vi "rcvr text files to formated csv files Main VI.vi"() -> ()   [LabVIEW 2011]
uses:
  <vilib>/Utility/file.llb/Read From Spreadsheet File (string).vi
panel:
  in  "leap year":enum16{"NON Leap Year", "Leap Year"}(ring)
  in  "Directories to scan for all rcvr files":path[](array[path])
  in  "forced Elevation offset\n(Must by negative number)":dbl=-3.3537 max=0.0 format="%.4g"
  in  "Grennich Offset":dbl=-8.0
  out "stop time":timestamp
  out "start time":timestamp
  out "# of files already done":i32
  out "# of files to convert":i32
  in  "first part of CSV file name (date will be added to end of file)":string
  in  "Directory to save new CSV files into":path
  # "Use -8 for Pacific standard time. Correct from UTM time to Local Standard Time.\nThere is a VI that corrects for DST. (Only good for 2011)"
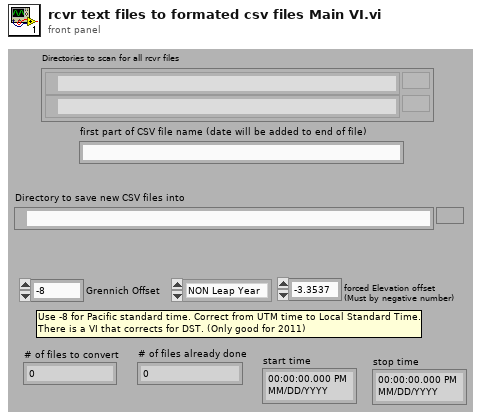
[diagram p1: front panel]
types:
  T1 = enum16{"open", "replace", "create", "open or create", "replace or create", "replace or create with confirmation"}
  T2 = cluster{"Time of NEMA":cluster{"Seconds":i32, "Minutes":i32, "Hours":i32}, "Lat-Long in Decimal Degrees":cluster{"Latitude (DD)":dbl, "Longitude (DD)":dbl}, "Point quality variables":cluster{"HDOP":dbl, "#Sats":dbl, "fixQuality":dbl}, "Elevations":cluster{"Elevation (Mean Sea Level)":dbl, "geodal separation":dbl, "Elevation (Height above Elipsode)":dbl}}
  T3 = cluster{"Latitude (DD)":dbl, "Longitude (DD)":dbl}
  T4 = cluster{"Seconds":i32, "Minutes":i32, "Hours":i32}
  T5 = typedef "LVDateTimeRec.ctl" = cluster{"fractional second":dbl, "second":i32, "minute":i32, "hour":i32, "day of month":i32, "month":i32, "year":i32, "day of week":i32, "day of year":i32, "DST":i32}
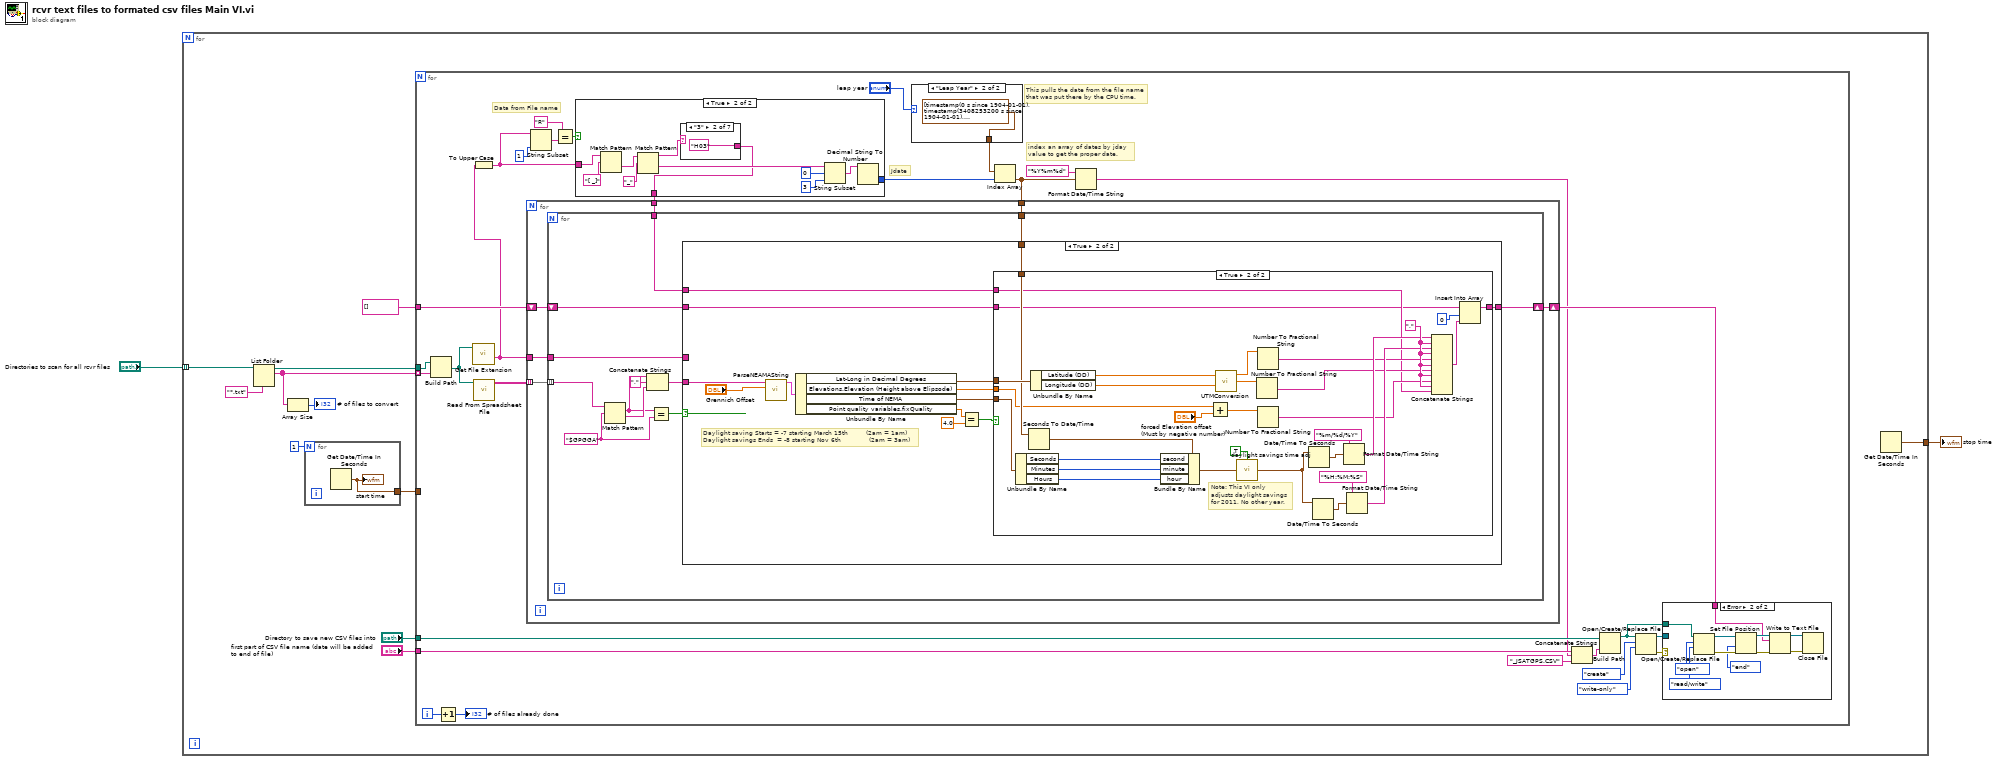
[diagram p0: block diagram]
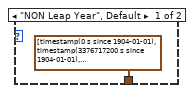
[diagram p2: hidden frame]
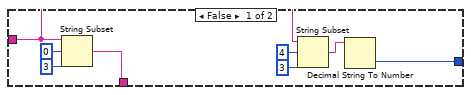
[diagram p3: hidden frame]
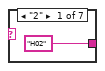
[diagram p4: hidden frame]
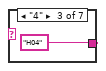
[diagram p5: hidden frame]
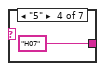
[diagram p6: hidden frame]
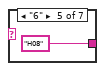
[diagram p7: hidden frame]
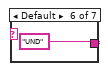
[diagram p8: hidden frame]
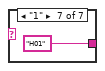
[diagram p9: hidden frame]
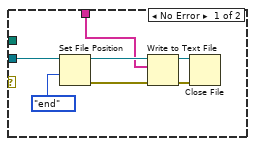
[diagram p10: hidden frame]
diagram:
  n1 = for {
    tunnel: [w4] -> w2
    tunnel: "Directories to scan for all rcvr files" -> [w3] mode=indexing
    n2 = List Folder(path=w3, pattern="*.txt") -> (path out=w12:path, filenames=w9:string[])  [unwired: 2 in, 2 out]
    n3 = Array Size(array=w9) -> (size(s)=→"# of files to convert":i32)
    n4 = for {
      N: 1 -> [_]
      tunnel: [w14] -> w6
      n5 = Get Date/Time In Seconds() -> (seconds since 1Jan1904=w14:timestamp)
      "start time" <- w14
    }
    n6 = for {
      tunnel: w12 -> [w44]
      tunnel: w9 -> [w43] mode=indexing
      tunnel: "Directory to save new CSV files into" -> [w39]
      tunnel: "first part of CSV file name (date will be added to end of file)" -> [w37]
      tunnel: string[] [] -> [w40]
      tunnel: w6 -> [_]
      i -> [w28]
      # "Jdate"
      # "This pulls the date from the file name\nthat was put there by the CPU time."
      # "Data from File name"
      # "index an array of dates by jday \nvalue to get the proper date."
      n7 = Build Path(base path=w44, name or relative path=w43) -> (appended path=w42:path)
      n8 = Increment(x=w28) -> (x+1=→"# of files already done":i32)
      n9 = call <vilib>:"Get File Extension.vi"("file"=w42) -> ("filename without extension"=w19:string)  [unwired: 7 in, 3 out]
      n10 = To Upper Case(1:w19) -> (0:w18:string)
      n11 = call-poly <vilib>:"Read From Spreadsheet File.vi"("file path (dialog if empty)"=w42) -> ("all rows"=w41:string[][])  [unwired: 6 in, 4 out]
      n12 = String Subset(string=w18, length (rest)=1 ("length (rest)")) -> (substring=w21:string)  [unwired: 1 in]
      n13 = Equal?(x="R", y=w21) -> (x = y?=w22:bool)
      n14 = case shown="True" w22 {
        tunnel: [w52 w58] -> w24
        tunnel: w18 -> [w48 w57]
        tunnel: [w47 w55] -> w16
        frame False {
          n15 = String Subset(string=w48, offset (0)=0, length (rest)=3 ("length (rest)")) -> (substring=w47:string)
          n16 = String Subset(string=w48, offset (0)=4, length (rest)=3 ("length (rest)")) -> (substring=w49:string)
          n17 = Decimal String To Number(string=w49) -> (number=w52:i32)  [unwired: 2 in, 1 out]
        }
        frame True {
          n18 = Match Pattern(string=w57, regular expression="[ _]") -> (after substring=w62:string)  [unwired: 1 in, 3 out]
          n19 = Match Pattern(string=w62, regular expression="_") -> (before substring=w56:string, after substring=w59:string)  [unwired: 1 in, 2 out]
          n20 = case shown="\"3\"" w56 {
            tunnel: ["H02" "H03" "H04" "H07" "H08" "UND" "H01"] -> w55
            frame "2" {
            }
            frame "3" {
            }
            frame "4" {
            }
            frame "5" {
            }
            frame "6" {
            }
            frame Default {
            }
            frame "1" {
            }
          }
          n21 = String Subset(string=w59, offset (0)=0, length (rest)=3 ("offset (0)")) -> (substring=w65:string)
          n22 = Decimal String To Number(string=w65) -> (number=w58:i32)  [unwired: 2 in, 1 out]
        }
      }
      n23 = case shown="\"Leap Year\"" "leap year" {
        tunnel: [timestamp[] [timestamp(0 s since 1904-01-01), timestamp(3376717200 s since 1904-01-01), timestamp(3376803600 s since 1904-01-01), timestamp(3376890000 s since 1904-01-01), timestamp(3376976400 s since 1904-01-01), timestamp(3377062800 s since 1904-01-01), timestamp(3377149200 s since 1904-01-01), timestamp(3377235600 s since 1904-01-01), timestamp(3377322000 s since 1904-01-01), timestamp(3377408400 s since 1904-01-01), timestamp(3377494800 s since 1904-01-01), timestamp(3377581200 s since 1904-01-01), timestamp(3377667600 s since 1904-01-01), timestamp(3377754000 s since 1904-01-01), timestamp(3377840400 s since 1904-01-01), timestamp(3377926800 s since 1904-01-01), timestamp(3378013200 s since 1904-01-01), timestamp(3378099600 s since 1904-01-01), timestamp(3378186000 s since 1904-01-01), timestamp(3378272400 s since 1904-01-01), timestamp(3378358800 s since 1904-01-01), timestamp(3378445200 s since 1904-01-01), timestamp(3378531600 s since 1904-01-01), timestamp(3378618000 s since 1904-01-01), timestamp(3378704400 s since 1904-01-01), timestamp(3378790800 s since 1904-01-01), timestamp(3378877200 s since 1904-01-01), timestamp(3378963600 s since 1904-01-01), timestamp(3379050000 s since 1904-01-01), timestamp(3379136400 s since 1904-01-01), timestamp(3379222800 s since 1904-01-01), timestamp(3379309200 s since 1904-01-01), timestamp(3379395600 s since 1904-01-01), timestamp(3379482000 s since 1904-01-01), timestamp(3379568400 s since 1904-01-01), timestamp(3379654800 s since 1904-01-01), timestamp(3379741200 s since 1904-01-01), timestamp(3379827600 s since 1904-01-01), timestamp(3379914000 s since 1904-01-01), timestamp(3380000400 s since 1904-01-01), timestamp(3380086800 s since 1904-01-01), timestamp(3380173200 s since 1904-01-01), timestamp(3380259600 s since 1904-01-01), timestamp(3380346000 s since 1904-01-01), timestamp(3380432400 s since 1904-01-01), timestamp(3380518800 s since 1904-01-01), timestamp(3380605200 s since 1904-01-01), timestamp(3380691600 s since 1904-01-01), timestamp(3380778000 s since 1904-01-01), timestamp(3380864400 s since 1904-01-01), timestamp(3380950800 s since 1904-01-01), timestamp(3381037200 s since 1904-01-01), timestamp(3381123600 s since 1904-01-01), timestamp(3381210000 s since 1904-01-01), timestamp(3381296400 s since 1904-01-01), timestamp(3381382800 s since 1904-01-01), timestamp(3381469200 s since 1904-01-01), timestamp(3381555600 s since 1904-01-01), timestamp(3381642000 s since 1904-01-01), timestamp(3381728400 s since 1904-01-01), timestamp(3381814800 s since 1904-01-01), timestamp(3381901200 s since 1904-01-01), timestamp(3381987600 s since 1904-01-01), timestamp(3382074000 s since 1904-01-01), timestamp(3382160400 s since 1904-01-01), timestamp(3382246800 s since 1904-01-01), timestamp(3382333200 s since 1904-01-01), timestamp(3382419600 s since 1904-01-01), timestamp(3382506000 s since 1904-01-01), timestamp(3382592400 s since 1904-01-01), timestamp(3382678800 s since 1904-01-01), timestamp(3382765200 s since 1904-01-01), timestamp(3382851600 s since 1904-01-01), timestamp(3382938000 s since 1904-01-01), timestamp(3383024400 s since 1904-01-01), timestamp(3383110800 s since 1904-01-01), timestamp(3383197200 s since 1904-01-01), timestamp(3383283600 s since 1904-01-01), timestamp(3383370000 s since 1904-01-01), timestamp(3383456400 s since 1904-01-01), timestamp(3383542800 s since 1904-01-01), timestamp(3383629200 s since 1904-01-01), timestamp(3383715600 s since 1904-01-01), timestamp(3383802000 s since 1904-01-01), timestamp(3383888400 s since 1904-01-01), timestamp(3383974800 s since 1904-01-01), timestamp(3384061200 s since 1904-01-01), timestamp(3384147600 s since 1904-01-01), timestamp(3384234000 s since 1904-01-01), timestamp(3384320400 s since 1904-01-01), timestamp(3384406800 s since 1904-01-01), timestamp(3384493200 s since 1904-01-01), timestamp(3384579600 s since 1904-01-01), timestamp(3384666000 s since 1904-01-01), timestamp(3384752400 s since 1904-01-01), timestamp(3384838800 s since 1904-01-01), timestamp(3384925200 s since 1904-01-01), timestamp(3385011600 s since 1904-01-01), timestamp(3385098000 s since 1904-01-01), timestamp(3385184400 s since 1904-01-01), timestamp(3385270800 s since 1904-01-01), timestamp(3385357200 s since 1904-01-01), timestamp(3385443600 s since 1904-01-01), timestamp(3385530000 s since 1904-01-01), timestamp(3385616400 s since 1904-01-01), timestamp(3385702800 s since 1904-01-01), timestamp(3385789200 s since 1904-01-01), timestamp(3385875600 s since 1904-01-01), timestamp(3385962000 s since 1904-01-01), timestamp(3386048400 s since 1904-01-01), timestamp(3386134800 s since 1904-01-01), timestamp(3386221200 s since 1904-01-01), timestamp(3386307600 s since 1904-01-01), timestamp(3386394000 s since 1904-01-01), timestamp(3386480400 s since 1904-01-01), timestamp(3386566800 s since 1904-01-01), timestamp(3386653200 s since 1904-01-01), timestamp(3386739600 s since 1904-01-01), timestamp(3386826000 s since 1904-01-01), timestamp(3386912400 s since 1904-01-01), timestamp(3386998800 s since 1904-01-01), timestamp(3387085200 s since 1904-01-01), timestamp(3387171600 s since 1904-01-01), timestamp(3387258000 s since 1904-01-01), timestamp(3387344400 s since 1904-01-01), timestamp(3387430800 s since 1904-01-01), timestamp(3387517200 s since 1904-01-01), timestamp(3387603600 s since 1904-01-01), timestamp(3387690000 s since 1904-01-01), timestamp(3387776400 s since 1904-01-01), timestamp(3387862800 s since 1904-01-01), timestamp(3387949200 s since 1904-01-01), timestamp(3388035600 s since 1904-01-01), timestamp(3388122000 s since 1904-01-01), timestamp(3388208400 s since 1904-01-01), timestamp(3388294800 s since 1904-01-01), timestamp(3388381200 s since 1904-01-01), timestamp(3388467600 s since 1904-01-01), timestamp(3388554000 s since 1904-01-01), timestamp(3388640400 s since 1904-01-01), timestamp(3388726800 s since 1904-01-01), timestamp(3388813200 s since 1904-01-01), timestamp(3388899600 s since 1904-01-01), timestamp(3388986000 s since 1904-01-01), timestamp(3389072400 s since 1904-01-01), timestamp(3389158800 s since 1904-01-01), timestamp(3389245200 s since 1904-01-01), timestamp(3389331600 s since 1904-01-01), timestamp(3389418000 s since 1904-01-01), timestamp(3389504400 s since 1904-01-01), timestamp(3389590800 s since 1904-01-01), timestamp(3389677200 s since 1904-01-01), timestamp(3389763600 s since 1904-01-01), timestamp(3389850000 s since 1904-01-01), timestamp(3389936400 s since 1904-01-01), timestamp(3390022800 s since 1904-01-01), timestamp(3390109200 s since 1904-01-01), timestamp(3390195600 s since 1904-01-01), timestamp(3390282000 s since 1904-01-01), timestamp(3390368400 s since 1904-01-01), timestamp(3390454800 s since 1904-01-01), timestamp(3390541200 s since 1904-01-01), timestamp(3390627600 s since 1904-01-01), timestamp(3390714000 s since 1904-01-01), timestamp(3390800400 s since 1904-01-01), timestamp(3390886800 s since 1904-01-01), timestamp(3390973200 s since 1904-01-01), timestamp(3391059600 s since 1904-01-01), timestamp(3391146000 s since 1904-01-01), timestamp(3391232400 s since 1904-01-01), timestamp(3391318800 s since 1904-01-01), timestamp(3391405200 s since 1904-01-01), timestamp(3391491600 s since 1904-01-01), timestamp(3391578000 s since 1904-01-01), timestamp(3391664400 s since 1904-01-01), timestamp(3391750800 s since 1904-01-01), timestamp(3391837200 s since 1904-01-01), timestamp(3391923600 s since 1904-01-01), timestamp(3392010000 s since 1904-01-01), timestamp(3392096400 s since 1904-01-01), timestamp(3392182800 s since 1904-01-01), timestamp(3392269200 s since 1904-01-01), timestamp(3392355600 s since 1904-01-01), timestamp(3392442000 s since 1904-01-01), timestamp(3392528400 s since 1904-01-01), timestamp(3392614800 s since 1904-01-01), timestamp(3392701200 s since 1904-01-01), timestamp(3392787600 s since 1904-01-01), timestamp(3392874000 s since 1904-01-01), timestamp(3392960400 s since 1904-01-01), timestamp(3393046800 s since 1904-01-01), timestamp(3393133200 s since 1904-01-01), timestamp(3393219600 s since 1904-01-01), timestamp(3393306000 s since 1904-01-01), timestamp(3393392400 s since 1904-01-01), timestamp(3393478800 s since 1904-01-01), timestamp(3393565200 s since 1904-01-01), timestamp(3393651600 s since 1904-01-01), timestamp(3393738000 s since 1904-01-01), timestamp(3393824400 s since 1904-01-01), timestamp(3393910800 s since 1904-01-01), timestamp(3393997200 s since 1904-01-01), timestamp(3394083600 s since 1904-01-01), timestamp(3394170000 s since 1904-01-01), timestamp(3394256400 s since 1904-01-01), timestamp(3394342800 s since 1904-01-01), timestamp(3394429200 s since 1904-01-01), timestamp(3394515600 s since 1904-01-01), timestamp(3394602000 s since 1904-01-01), timestamp(3394688400 s since 1904-01-01), timestamp(3394774800 s since 1904-01-01), timestamp(3394861200 s since 1904-01-01), timestamp(3394947600 s since 1904-01-01), timestamp(3395034000 s since 1904-01-01), timestamp(3395120400 s since 1904-01-01), timestamp(3395206800 s since 1904-01-01), timestamp(3395293200 s since 1904-01-01), timestamp(3395379600 s since 1904-01-01), timestamp(3395466000 s since 1904-01-01), timestamp(3395552400 s since 1904-01-01), timestamp(3395638800 s since 1904-01-01), timestamp(3395725200 s since 1904-01-01), timestamp(3395811600 s since 1904-01-01), timestamp(3395898000 s since 1904-01-01), timestamp(3395984400 s since 1904-01-01), timestamp(3396070800 s since 1904-01-01), timestamp(3396157200 s since 1904-01-01), timestamp(3396243600 s since 1904-01-01), timestamp(3396330000 s since 1904-01-01), timestamp(3396416400 s since 1904-01-01), timestamp(3396502800 s since 1904-01-01), timestamp(3396589200 s since 1904-01-01), timestamp(3396675600 s since 1904-01-01), timestamp(3396762000 s since 1904-01-01), timestamp(3396848400 s since 1904-01-01), timestamp(3396934800 s since 1904-01-01), timestamp(3397021200 s since 1904-01-01), timestamp(3397107600 s since 1904-01-01), timestamp(3397194000 s since 1904-01-01), timestamp(3397280400 s since 1904-01-01), timestamp(3397366800 s since 1904-01-01), timestamp(3397453200 s since 1904-01-01), timestamp(3397539600 s since 1904-01-01), timestamp(3397626000 s since 1904-01-01), timestamp(3397712400 s since 1904-01-01), timestamp(3397798800 s since 1904-01-01), timestamp(3397885200 s since 1904-01-01), timestamp(3397971600 s since 1904-01-01), timestamp(3398058000 s since 1904-01-01), timestamp(3398144400 s since 1904-01-01), timestamp(3398230800 s since 1904-01-01), timestamp(3398317200 s since 1904-01-01), timestamp(3398403600 s since 1904-01-01), timestamp(3398490000 s since 1904-01-01), timestamp(3398576400 s since 1904-01-01), timestamp(3398662800 s since 1904-01-01), timestamp(3398749200 s since 1904-01-01), timestamp(3398835600 s since 1904-01-01), timestamp(3398922000 s since 1904-01-01), timestamp(3399008400 s since 1904-01-01), timestamp(3399094800 s since 1904-01-01), timestamp(3399181200 s since 1904-01-01), timestamp(3399267600 s since 1904-01-01), timestamp(3399354000 s since 1904-01-01), timestamp(3399440400 s since 1904-01-01), timestamp(3399526800 s since 1904-01-01), timestamp(3399613200 s since 1904-01-01), timestamp(3399699600 s since 1904-01-01), timestamp(3399786000 s since 1904-01-01), timestamp(3399872400 s since 1904-01-01), timestamp(3399958800 s since 1904-01-01), timestamp(3400045200 s since 1904-01-01), timestamp(3400131600 s since 1904-01-01), timestamp(3400218000 s since 1904-01-01), timestamp(3400304400 s since 1904-01-01), timestamp(3400390800 s since 1904-01-01), timestamp(3400477200 s since 1904-01-01), timestamp(3400563600 s since 1904-01-01), timestamp(3400650000 s since 1904-01-01), timestamp(3400736400 s since 1904-01-01), timestamp(3400822800 s since 1904-01-01), timestamp(3400909200 s since 1904-01-01), timestamp(3400995600 s since 1904-01-01), timestamp(3401082000 s since 1904-01-01), timestamp(3401168400 s since 1904-01-01), timestamp(3401254800 s since 1904-01-01), timestamp(3401341200 s since 1904-01-01), timestamp(3401427600 s since 1904-01-01), timestamp(3401514000 s since 1904-01-01), timestamp(3401600400 s since 1904-01-01), timestamp(3401686800 s since 1904-01-01), timestamp(3401773200 s since 1904-01-01), timestamp(3401859600 s since 1904-01-01), timestamp(3401946000 s since 1904-01-01), timestamp(3402032400 s since 1904-01-01), timestamp(3402118800 s since 1904-01-01), timestamp(3402205200 s since 1904-01-01), timestamp(3402291600 s since 1904-01-01), timestamp(3402378000 s since 1904-01-01), timestamp(3402464400 s since 1904-01-01), timestamp(3402550800 s since 1904-01-01), timestamp(3402637200 s since 1904-01-01), timestamp(3402723600 s since 1904-01-01), timestamp(3402810000 s since 1904-01-01), timestamp(3402896400 s since 1904-01-01), timestamp(3402982800 s since 1904-01-01), timestamp(3403069200 s since 1904-01-01), timestamp(3403155600 s since 1904-01-01), timestamp(3403242000 s since 1904-01-01), timestamp(3403328400 s since 1904-01-01), timestamp(3403414800 s since 1904-01-01), timestamp(3403501200 s since 1904-01-01), timestamp(3403587600 s since 1904-01-01), timestamp(3403674000 s since 1904-01-01), timestamp(3403760400 s since 1904-01-01), timestamp(3403846800 s since 1904-01-01), timestamp(3403933200 s since 1904-01-01), timestamp(3404019600 s since 1904-01-01), timestamp(3404106000 s since 1904-01-01), timestamp(3404192400 s since 1904-01-01), timestamp(3404278800 s since 1904-01-01), timestamp(3404365200 s since 1904-01-01), timestamp(3404451600 s since 1904-01-01), timestamp(3404538000 s since 1904-01-01), timestamp(3404624400 s since 1904-01-01), timestamp(3404710800 s since 1904-01-01), timestamp(3404797200 s since 1904-01-01), timestamp(3404883600 s since 1904-01-01), timestamp(3404970000 s since 1904-01-01), timestamp(3405056400 s since 1904-01-01), timestamp(3405142800 s since 1904-01-01), timestamp(3405229200 s since 1904-01-01), timestamp(3405315600 s since 1904-01-01), timestamp(3405402000 s since 1904-01-01), timestamp(3405488400 s since 1904-01-01), timestamp(3405574800 s since 1904-01-01), timestamp(3405661200 s since 1904-01-01), timestamp(3405747600 s since 1904-01-01), timestamp(3405834000 s since 1904-01-01), timestamp(3405920400 s since 1904-01-01), timestamp(3406006800 s since 1904-01-01), timestamp(3406093200 s since 1904-01-01), timestamp(3406179600 s since 1904-01-01), timestamp(3406266000 s since 1904-01-01), timestamp(3406352400 s since 1904-01-01), timestamp(3406438800 s since 1904-01-01), timestamp(3406525200 s since 1904-01-01), timestamp(3406611600 s since 1904-01-01), timestamp(3406698000 s since 1904-01-01), timestamp(3406784400 s since 1904-01-01), timestamp(3406870800 s since 1904-01-01), timestamp(3406957200 s since 1904-01-01), timestamp(3407043600 s since 1904-01-01), timestamp(3407130000 s since 1904-01-01), timestamp(3407216400 s since 1904-01-01), timestamp(3407302800 s since 1904-01-01), timestamp(3407389200 s since 1904-01-01), timestamp(3407475600 s since 1904-01-01), timestamp(3407562000 s since 1904-01-01), timestamp(3407648400 s since 1904-01-01), timestamp(3407734800 s since 1904-01-01), timestamp(3407821200 s since 1904-01-01), timestamp(3407907600 s since 1904-01-01), timestamp(3407994000 s since 1904-01-01), timestamp(3408080400 s since 1904-01-01), timestamp(3408166800 s since 1904-01-01)] ("Julian day to calander day non leap year (index = Julian day)") timestamp[] [timestamp(0 s since 1904-01-01), timestamp(3408253200 s since 1904-01-01), timestamp(3408339600 s since 1904-01-01), timestamp(3408426000 s since 1904-01-01), timestamp(3408512400 s since 1904-01-01), timestamp(3408598800 s since 1904-01-01), timestamp(3408685200 s since 1904-01-01), timestamp(3408771600 s since 1904-01-01), timestamp(3408858000 s since 1904-01-01), timestamp(3408944400 s since 1904-01-01), timestamp(3409030800 s since 1904-01-01), timestamp(3409117200 s since 1904-01-01), timestamp(3409203600 s since 1904-01-01), timestamp(3409290000 s since 1904-01-01), timestamp(3409376400 s since 1904-01-01), timestamp(3409462800 s since 1904-01-01), timestamp(3409549200 s since 1904-01-01), timestamp(3409635600 s since 1904-01-01), timestamp(3409722000 s since 1904-01-01), timestamp(3409808400 s since 1904-01-01), timestamp(3409894800 s since 1904-01-01), timestamp(3409981200 s since 1904-01-01), timestamp(3410067600 s since 1904-01-01), timestamp(3410154000 s since 1904-01-01), timestamp(3410240400 s since 1904-01-01), timestamp(3410326800 s since 1904-01-01), timestamp(3410413200 s since 1904-01-01), timestamp(3410499600 s since 1904-01-01), timestamp(3410586000 s since 1904-01-01), timestamp(3410672400 s since 1904-01-01), timestamp(3410758800 s since 1904-01-01), timestamp(3410845200 s since 1904-01-01), timestamp(3410931600 s since 1904-01-01), timestamp(3411018000 s since 1904-01-01), timestamp(3411104400 s since 1904-01-01), timestamp(3411190800 s since 1904-01-01), timestamp(3411277200 s since 1904-01-01), timestamp(3411363600 s since 1904-01-01), timestamp(3411450000 s since 1904-01-01), timestamp(3411536400 s since 1904-01-01), timestamp(3411622800 s since 1904-01-01), timestamp(3411709200 s since 1904-01-01), timestamp(3411795600 s since 1904-01-01), timestamp(3411882000 s since 1904-01-01), timestamp(3411968400 s since 1904-01-01), timestamp(3412054800 s since 1904-01-01), timestamp(3412141200 s since 1904-01-01), timestamp(3412227600 s since 1904-01-01), timestamp(3412314000 s since 1904-01-01), timestamp(3412400400 s since 1904-01-01), timestamp(3412486800 s since 1904-01-01), timestamp(3412573200 s since 1904-01-01), timestamp(3412659600 s since 1904-01-01), timestamp(3412746000 s since 1904-01-01), timestamp(3412832400 s since 1904-01-01), timestamp(3412918800 s since 1904-01-01), timestamp(3413005200 s since 1904-01-01), timestamp(3413091600 s since 1904-01-01), timestamp(3413178000 s since 1904-01-01), timestamp(3413264400 s since 1904-01-01), timestamp(3413350800 s since 1904-01-01), timestamp(3413437200 s since 1904-01-01), timestamp(3413523600 s since 1904-01-01), timestamp(3413610000 s since 1904-01-01), timestamp(3413696400 s since 1904-01-01), timestamp(3413782800 s since 1904-01-01), timestamp(3413869200 s since 1904-01-01), timestamp(3413955600 s since 1904-01-01), timestamp(3414042000 s since 1904-01-01), timestamp(3414128400 s since 1904-01-01), timestamp(3414214800 s since 1904-01-01), timestamp(3414301200 s since 1904-01-01), timestamp(3414387600 s since 1904-01-01), timestamp(3414474000 s since 1904-01-01), timestamp(3414560400 s since 1904-01-01), timestamp(3414646800 s since 1904-01-01), timestamp(3414733200 s since 1904-01-01), timestamp(3414819600 s since 1904-01-01), timestamp(3414906000 s since 1904-01-01), timestamp(3414992400 s since 1904-01-01), timestamp(3415078800 s since 1904-01-01), timestamp(3415165200 s since 1904-01-01), timestamp(3415251600 s since 1904-01-01), timestamp(3415338000 s since 1904-01-01), timestamp(3415424400 s since 1904-01-01), timestamp(3415510800 s since 1904-01-01), timestamp(3415597200 s since 1904-01-01), timestamp(3415683600 s since 1904-01-01), timestamp(3415770000 s since 1904-01-01), timestamp(3415856400 s since 1904-01-01), timestamp(3415942800 s since 1904-01-01), timestamp(3416029200 s since 1904-01-01), timestamp(3416115600 s since 1904-01-01), timestamp(3416202000 s since 1904-01-01), timestamp(3416288400 s since 1904-01-01), timestamp(3416374800 s since 1904-01-01), timestamp(3416461200 s since 1904-01-01), timestamp(3416547600 s since 1904-01-01), timestamp(3416634000 s since 1904-01-01), timestamp(3416720400 s since 1904-01-01), timestamp(3416806800 s since 1904-01-01), timestamp(3416893200 s since 1904-01-01), timestamp(3416979600 s since 1904-01-01), timestamp(3417066000 s since 1904-01-01), timestamp(3417152400 s since 1904-01-01), timestamp(3417238800 s since 1904-01-01), timestamp(3417325200 s since 1904-01-01), timestamp(3417411600 s since 1904-01-01), timestamp(3417498000 s since 1904-01-01), timestamp(3417584400 s since 1904-01-01), timestamp(3417670800 s since 1904-01-01), timestamp(3417757200 s since 1904-01-01), timestamp(3417843600 s since 1904-01-01), timestamp(3417930000 s since 1904-01-01), timestamp(3418016400 s since 1904-01-01), timestamp(3418102800 s since 1904-01-01), timestamp(3418189200 s since 1904-01-01), timestamp(3418275600 s since 1904-01-01), timestamp(3418362000 s since 1904-01-01), timestamp(3418448400 s since 1904-01-01), timestamp(3418534800 s since 1904-01-01), timestamp(3418621200 s since 1904-01-01), timestamp(3418707600 s since 1904-01-01), timestamp(3418794000 s since 1904-01-01), timestamp(3418880400 s since 1904-01-01), timestamp(3418966800 s since 1904-01-01), timestamp(3419053200 s since 1904-01-01), timestamp(3419139600 s since 1904-01-01), timestamp(3419226000 s since 1904-01-01), timestamp(3419312400 s since 1904-01-01), timestamp(3419398800 s since 1904-01-01), timestamp(3419485200 s since 1904-01-01), timestamp(3419571600 s since 1904-01-01), timestamp(3419658000 s since 1904-01-01), timestamp(3419744400 s since 1904-01-01), timestamp(3419830800 s since 1904-01-01), timestamp(3419917200 s since 1904-01-01), timestamp(3420003600 s since 1904-01-01), timestamp(3420090000 s since 1904-01-01), timestamp(3420176400 s since 1904-01-01), timestamp(3420262800 s since 1904-01-01), timestamp(3420349200 s since 1904-01-01), timestamp(3420435600 s since 1904-01-01), timestamp(3420522000 s since 1904-01-01), timestamp(3420608400 s since 1904-01-01), timestamp(3420694800 s since 1904-01-01), timestamp(3420781200 s since 1904-01-01), timestamp(3420867600 s since 1904-01-01), timestamp(3420954000 s since 1904-01-01), timestamp(3421040400 s since 1904-01-01), timestamp(3421126800 s since 1904-01-01), timestamp(3421213200 s since 1904-01-01), timestamp(3421299600 s since 1904-01-01), timestamp(3421386000 s since 1904-01-01), timestamp(3421472400 s since 1904-01-01), timestamp(3421558800 s since 1904-01-01), timestamp(3421645200 s since 1904-01-01), timestamp(3421731600 s since 1904-01-01), timestamp(3421818000 s since 1904-01-01), timestamp(3421904400 s since 1904-01-01), timestamp(3421990800 s since 1904-01-01), timestamp(3422077200 s since 1904-01-01), timestamp(3422163600 s since 1904-01-01), timestamp(3422250000 s since 1904-01-01), timestamp(3422336400 s since 1904-01-01), timestamp(3422422800 s since 1904-01-01), timestamp(3422509200 s since 1904-01-01), timestamp(3422595600 s since 1904-01-01), timestamp(3422682000 s since 1904-01-01), timestamp(3422768400 s since 1904-01-01), timestamp(3422854800 s since 1904-01-01), timestamp(3422941200 s since 1904-01-01), timestamp(3423027600 s since 1904-01-01), timestamp(3423114000 s since 1904-01-01), timestamp(3423200400 s since 1904-01-01), timestamp(3423286800 s since 1904-01-01), timestamp(3423373200 s since 1904-01-01), timestamp(3423459600 s since 1904-01-01), timestamp(3423546000 s since 1904-01-01), timestamp(3423632400 s since 1904-01-01), timestamp(3423718800 s since 1904-01-01), timestamp(3423805200 s since 1904-01-01), timestamp(3423891600 s since 1904-01-01), timestamp(3423978000 s since 1904-01-01), timestamp(3424064400 s since 1904-01-01), timestamp(3424150800 s since 1904-01-01), timestamp(3424237200 s since 1904-01-01), timestamp(3424323600 s since 1904-01-01), timestamp(3424410000 s since 1904-01-01), timestamp(3424496400 s since 1904-01-01), timestamp(3424582800 s since 1904-01-01), timestamp(3424669200 s since 1904-01-01), timestamp(3424755600 s since 1904-01-01), timestamp(3424842000 s since 1904-01-01), timestamp(3424928400 s since 1904-01-01), timestamp(3425014800 s since 1904-01-01), timestamp(3425101200 s since 1904-01-01), timestamp(3425187600 s since 1904-01-01), timestamp(3425274000 s since 1904-01-01), timestamp(3425360400 s since 1904-01-01), timestamp(3425446800 s since 1904-01-01), timestamp(3425533200 s since 1904-01-01), timestamp(3425619600 s since 1904-01-01), timestamp(3425706000 s since 1904-01-01), timestamp(3425792400 s since 1904-01-01), timestamp(3425878800 s since 1904-01-01), timestamp(3425965200 s since 1904-01-01), timestamp(3426051600 s since 1904-01-01), timestamp(3426138000 s since 1904-01-01), timestamp(3426224400 s since 1904-01-01), timestamp(3426310800 s since 1904-01-01), timestamp(3426397200 s since 1904-01-01), timestamp(3426483600 s since 1904-01-01), timestamp(3426570000 s since 1904-01-01), timestamp(3426656400 s since 1904-01-01), timestamp(3426742800 s since 1904-01-01), timestamp(3426829200 s since 1904-01-01), timestamp(3426915600 s since 1904-01-01), timestamp(3427002000 s since 1904-01-01), timestamp(3427088400 s since 1904-01-01), timestamp(3427174800 s since 1904-01-01), timestamp(3427261200 s since 1904-01-01), timestamp(3427347600 s since 1904-01-01), timestamp(3427434000 s since 1904-01-01), timestamp(3427520400 s since 1904-01-01), timestamp(3427606800 s since 1904-01-01), timestamp(3427693200 s since 1904-01-01), timestamp(3427779600 s since 1904-01-01), timestamp(3427866000 s since 1904-01-01), timestamp(3427952400 s since 1904-01-01), timestamp(3428038800 s since 1904-01-01), timestamp(3428125200 s since 1904-01-01), timestamp(3428211600 s since 1904-01-01), timestamp(3428298000 s since 1904-01-01), timestamp(3428384400 s since 1904-01-01), timestamp(3428470800 s since 1904-01-01), timestamp(3428557200 s since 1904-01-01), timestamp(3428643600 s since 1904-01-01), timestamp(3428730000 s since 1904-01-01), timestamp(3428816400 s since 1904-01-01), timestamp(3428902800 s since 1904-01-01), timestamp(3428989200 s since 1904-01-01), timestamp(3429075600 s since 1904-01-01), timestamp(3429162000 s since 1904-01-01), timestamp(3429248400 s since 1904-01-01), timestamp(3429334800 s since 1904-01-01), timestamp(3429421200 s since 1904-01-01), timestamp(3429507600 s since 1904-01-01), timestamp(3429594000 s since 1904-01-01), timestamp(3429680400 s since 1904-01-01), timestamp(3429766800 s since 1904-01-01), timestamp(3429853200 s since 1904-01-01), timestamp(3429939600 s since 1904-01-01), timestamp(3430026000 s since 1904-01-01), timestamp(3430112400 s since 1904-01-01), timestamp(3430198800 s since 1904-01-01), timestamp(3430285200 s since 1904-01-01), timestamp(3430371600 s since 1904-01-01), timestamp(3430458000 s since 1904-01-01), timestamp(3430544400 s since 1904-01-01), timestamp(3430630800 s since 1904-01-01), timestamp(3430717200 s since 1904-01-01), timestamp(3430803600 s since 1904-01-01), timestamp(3430890000 s since 1904-01-01), timestamp(3430976400 s since 1904-01-01), timestamp(3431062800 s since 1904-01-01), timestamp(3431149200 s since 1904-01-01), timestamp(3431235600 s since 1904-01-01), timestamp(3431322000 s since 1904-01-01), timestamp(3431408400 s since 1904-01-01), timestamp(3431494800 s since 1904-01-01), timestamp(3431581200 s since 1904-01-01), timestamp(3431667600 s since 1904-01-01), timestamp(3431754000 s since 1904-01-01), timestamp(3431840400 s since 1904-01-01), timestamp(3431926800 s since 1904-01-01), timestamp(3432013200 s since 1904-01-01), timestamp(3432099600 s since 1904-01-01), timestamp(3432186000 s since 1904-01-01), timestamp(3432272400 s since 1904-01-01), timestamp(3432358800 s since 1904-01-01), timestamp(3432445200 s since 1904-01-01), timestamp(3432531600 s since 1904-01-01), timestamp(3432618000 s since 1904-01-01), timestamp(3432704400 s since 1904-01-01), timestamp(3432790800 s since 1904-01-01), timestamp(3432877200 s since 1904-01-01), timestamp(3432963600 s since 1904-01-01), timestamp(3433050000 s since 1904-01-01), timestamp(3433136400 s since 1904-01-01), timestamp(3433222800 s since 1904-01-01), timestamp(3433309200 s since 1904-01-01), timestamp(3433395600 s since 1904-01-01), timestamp(3433482000 s since 1904-01-01), timestamp(3433568400 s since 1904-01-01), timestamp(3433654800 s since 1904-01-01), timestamp(3433741200 s since 1904-01-01), timestamp(3433827600 s since 1904-01-01), timestamp(3433914000 s since 1904-01-01), timestamp(3434000400 s since 1904-01-01), timestamp(3434086800 s since 1904-01-01), timestamp(3434173200 s since 1904-01-01), timestamp(3434259600 s since 1904-01-01), timestamp(3434346000 s since 1904-01-01), timestamp(3434432400 s since 1904-01-01), timestamp(3434518800 s since 1904-01-01), timestamp(3434605200 s since 1904-01-01), timestamp(3434691600 s since 1904-01-01), timestamp(3434778000 s since 1904-01-01), timestamp(3434864400 s since 1904-01-01), timestamp(3434950800 s since 1904-01-01), timestamp(3435037200 s since 1904-01-01), timestamp(3435123600 s since 1904-01-01), timestamp(3435210000 s since 1904-01-01), timestamp(3435296400 s since 1904-01-01), timestamp(3435382800 s since 1904-01-01), timestamp(3435469200 s since 1904-01-01), timestamp(3435555600 s since 1904-01-01), timestamp(3435642000 s since 1904-01-01), timestamp(3435728400 s since 1904-01-01), timestamp(3435814800 s since 1904-01-01), timestamp(3435901200 s since 1904-01-01), timestamp(3435987600 s since 1904-01-01), timestamp(3436074000 s since 1904-01-01), timestamp(3436160400 s since 1904-01-01), timestamp(3436246800 s since 1904-01-01), timestamp(3436333200 s since 1904-01-01), timestamp(3436419600 s since 1904-01-01), timestamp(3436506000 s since 1904-01-01), timestamp(3436592400 s since 1904-01-01), timestamp(3436678800 s since 1904-01-01), timestamp(3436765200 s since 1904-01-01), timestamp(3436851600 s since 1904-01-01), timestamp(3436938000 s since 1904-01-01), timestamp(3437024400 s since 1904-01-01), timestamp(3437110800 s since 1904-01-01), timestamp(3437197200 s since 1904-01-01), timestamp(3437283600 s since 1904-01-01), timestamp(3437370000 s since 1904-01-01), timestamp(3437456400 s since 1904-01-01), timestamp(3437542800 s since 1904-01-01), timestamp(3437629200 s since 1904-01-01), timestamp(3437715600 s since 1904-01-01), timestamp(3437802000 s since 1904-01-01), timestamp(3437888400 s since 1904-01-01), timestamp(3437974800 s since 1904-01-01), timestamp(3438061200 s since 1904-01-01), timestamp(3438147600 s since 1904-01-01), timestamp(3438234000 s since 1904-01-01), timestamp(3438320400 s since 1904-01-01), timestamp(3438406800 s since 1904-01-01), timestamp(3438493200 s since 1904-01-01), timestamp(3438579600 s since 1904-01-01), timestamp(3438666000 s since 1904-01-01), timestamp(3438752400 s since 1904-01-01), timestamp(3438838800 s since 1904-01-01), timestamp(3438925200 s since 1904-01-01), timestamp(3439011600 s since 1904-01-01), timestamp(3439098000 s since 1904-01-01), timestamp(3439184400 s since 1904-01-01), timestamp(3439270800 s since 1904-01-01), timestamp(3439357200 s since 1904-01-01), timestamp(3439443600 s since 1904-01-01), timestamp(3439530000 s since 1904-01-01), timestamp(3439616400 s since 1904-01-01), timestamp(3439702800 s since 1904-01-01), timestamp(3439789200 s since 1904-01-01)] ("2012 2")] -> w32
        frame "NON Leap Year", Default {
        }
        frame "Leap Year" {
        }
      }
      n24 = Index Array(array=w32, index=w24) -> (element=w27:timestamp)
      n25 = for {
        tunnel: w41 -> [w95] mode=indexing
        tunnel: w19 -> [w96]
        shift-right: [w93] -> w31
        shift-left: w40 -> [w94]
        tunnel: w27 -> [w92]
        tunnel: w16 -> [w91]
        n26 = for {
          tunnel: w96 -> [w108]
          tunnel: w95 -> [w103] mode=indexing
          shift-right: [w106] -> w93
          shift-left: w94 -> [w107]
          tunnel: w92 -> [w105]
          tunnel: w91 -> [w97]
          w102 = "$GPGGA" ("y")
          n27 = Match Pattern(string=w103, regular expression=w102) -> (match substring=w98:string, after substring=w100:string)  [unwired: 1 in, 2 out]
          n28 = Concatenate Strings(w98, "," ("string"), w100) -> (w99:string)
          n29 = Equal?(x=w98, y=w102) -> (x = y?=w104:bool)
          n30 = case shown="True" w104 {
            tunnel: w108 -> [_ _]
            tunnel: w99 -> [_ w120]
            tunnel: w107 -> [w109 w116]
            tunnel: [w109 w117] -> w106
            tunnel: w105 -> [_ w115]
            tunnel: w97 -> [_ w110]
            frame False {
            }
            frame True {
              # "Daylight saving Starts = -7 starting March 15th         (2am = 1am)\nDaylight savings Ends  = -8 starting Nov 6th              (2am = 3am)"
              n31 = call "ParseNEAMAString.vi"("Grennich Offset"="Grennich Offset", "String In (NEAMA GGA)"=w120) -> ("NEMA string capture variables Out"=w122:T2)  [unwired: 6 in, 1 out]
              n32 = Unbundle By Name(w122) -> ("Lat-Long in Decimal Degrees"=w121:T3, "Elevations.Elevation (Height above Elipsode)"=w119:dbl, "Time of NEMA"=w118:T4, "Point quality variables.fixQuality"=w114:dbl)
              n33 = Equal?(x=w114, y=4.0) -> (x = y?=w112:bool)
              n34 = case shown="True" w112 {
                tunnel: w121 -> [_ w155]
                tunnel: w119 -> [_ w128]
                tunnel: w118 -> [_ w152]
                tunnel: [w123 w137] -> w117
                tunnel: w116 -> [w123 w136]
                tunnel: w115 -> [_ w151]
                tunnel: w110 -> [_ w138]
                frame False {
                }
                frame True {
                  w150 = ","
                  # "Note: This VI only \nadjusts daylight savings\nfor 2011, No other year."
                  n35 = Unbundle By Name(w152) -> ("Seconds"=w132:i32, "Minutes"=w131:i32, "Hours"=w130:i32)
                  n36 = Seconds To Date/Time(time stamp (now)=w151) -> (date time rec=w133:T5)  [unwired: 1 in]
                  n37 = Unbundle By Name(w155) -> ("Latitude (DD)"=w154:dbl, "Longitude (DD)"=w153:dbl)
                  n38 = Bundle By Name(cluster=w133, "second"=w132, "minute"=w131, "hour"=w130) -> (w126:T5)
                  n39 = Add(x=w128, y="forced Elevation offset\n(Must by negative number)") -> (x+y=w129:dbl)
                  n40 = call "UTMConversion.vi"("Lattitude"=w154, "Longitude"=w153) -> ("Easting"=w146:dbl, "Northing"=w147:dbl)  [unwired: 1 out]
                  n41 = call "daylight savings time adj.vi"("Apply daylight savings time"=TRUE, "Date Time (IN)"=w126) -> ("Date Time (out)"=w125:T5)  [unwired: 13 in]
                  n42 = Number To Fractional String(number=w147) -> (F-format string=w139:string)  [unwired: 3 in]
                  n43 = Number To Fractional String(number=w146) -> (F-format string=w140:string)  [unwired: 3 in]
                  n44 = Number To Fractional String(number=w129) -> (F-format string=w141:string)  [unwired: 3 in]
                  n45 = Date/Time To Seconds(2:w125) -> (0:w149:timestamp)  [unwired: 1 in]
                  n46 = Date/Time To Seconds(2:w125) -> (0:w144:timestamp)  [unwired: 1 in]
                  n47 = Format Date/Time String(time format string (%c)="%m/%d/%Y", seconds (now)=w149) -> (date/time string=w143:string)  [unwired: 1 in]
                  n48 = Format Date/Time String(time format string (%c)="%H:%M:%S", seconds (now)=w144) -> (date/time string=w142:string)  [unwired: 1 in]
                  n49 = Concatenate Strings(w143, w150, w142, w150, w140, w150, w139, w150, w141, w150, w138) -> (w134:string)
                  n50 = Insert Into Array(array=w136, index=0, new element=w134) -> (w137:string[])
                }
              }
            }
          }
        }
      }
      n51 = Format Date/Time String(time format string (%c)="%Y%m%d", seconds (now)=w27) -> (date/time string=w26:string)  [unwired: 1 in]
      n52 = Concatenate Strings(w37, w26, "_JSATGPS.CSV" ("string")) -> (w38:string)
      n53 = Build Path(base path=w39, name or relative path=w38) -> (appended path=w29:path)
      n54 = Open/Create/Replace File(file path (use dialog)=w29, operation (0:open)=T1."create", access (0:read/write)=enum16{"read/write", "read-only", "write-only"}."write-only") -> (refnum out=w33:refnum<file>, error out=w30:errorcluster)  [unwired: 3 in, 1 out]
      n55 = case shown="Error" w30 {
        tunnel: w33 -> [w77 _]
        tunnel: w31 -> [w73 w80]
        tunnel: w29 -> [_ w90]
        frame No Error {
          n56 = Set File Position(refnum=w77, from (0:start)=enum16{"start", "end", "current"}."end") -> (refnum out=w75:refnum<file>, error out=w74:errorcluster)  [unwired: 2 in]
          n57 = Write to Text File(file (use dialog)=w75, text=w73, error in=w74) -> (refnum out=w78:refnum<file>, error out=w79:errorcluster)  [unwired: 1 in, 1 out]
          n58 = Close File(refnum=w78, error in=w79) -> ()  [unwired: 2 out]
        }
        frame Error {
          n59 = Open/Create/Replace File(file path (use dialog)=w90, operation (0:open)=T1."open", access (0:read/write)=enum16{"read/write", "read-only", "write-only"}."read/write") -> (refnum out=w84:refnum<file>, error out=w85:errorcluster)  [unwired: 3 in, 1 out]
          n60 = Set File Position(refnum=w84, from (0:start)=enum16{"start", "end", "current"}."end", error in=w85) -> (refnum out=w82:refnum<file>, error out=w81:errorcluster)  [unwired: 1 in]
          n61 = Write to Text File(file (use dialog)=w82, text=w80, error in=w81) -> (refnum out=w86:refnum<file>, error out=w87:errorcluster)  [unwired: 1 in, 1 out]
          n62 = Close File(refnum=w86, error in=w87) -> ()  [unwired: 2 out]
        }
      }
    }
    n63 = Get Date/Time In Seconds() -> (seconds since 1Jan1904=w4:timestamp)
  }
  "stop time" <- w2
